vi "Convert Binary to TSV.vi"(8 "This VI":refnum<vi>, 11 "TDMS DataFile Name":path) -> ()   [LabVIEW 2023]
uses:
  User_Vi/Settings.vi
panel:
  out "error out 2":errorcluster
  out "error out":errorcluster
  out "Save a copy of the Binary Data File":bool
  out "PointsPerRow":u64
  out "NumberOfRowstoSave":i16
  out "ApproxBytes":dbl
  out "Save File Path":path
  out "Save Channels Separatly":bool
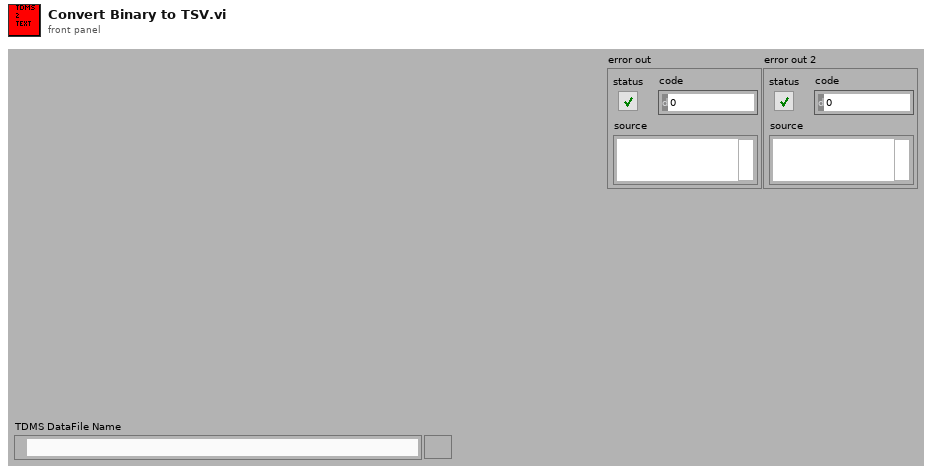
[diagram p1: front panel]
types:
  T1 = enum16{"open", "open or create", "create or replace", "create", "open (read-only)"}
  T2 = enum16{"open", "replace", "create", "open or create", "replace or create", "replace or create with confirmation"}
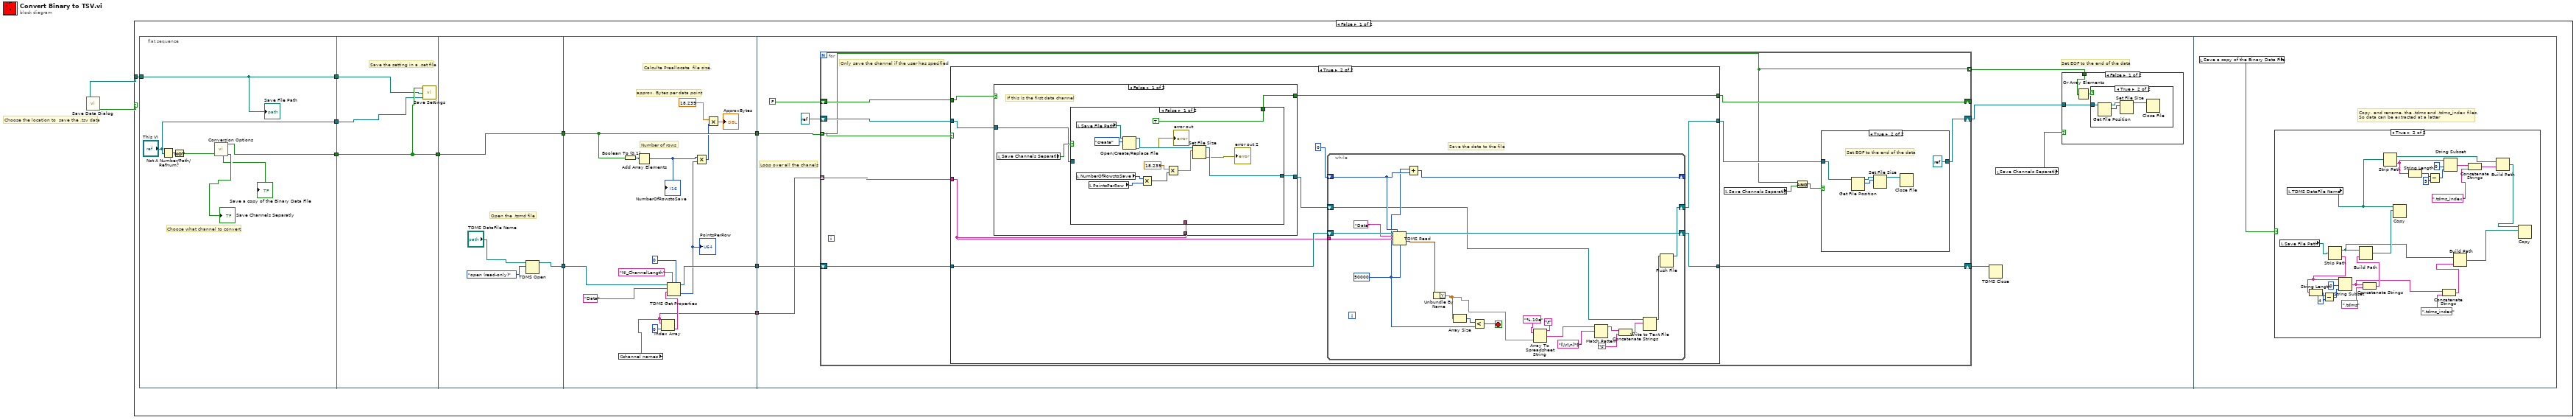
[diagram p0: block diagram]
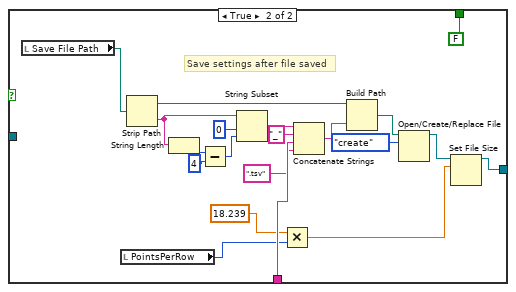
[diagram p6: hidden frame]
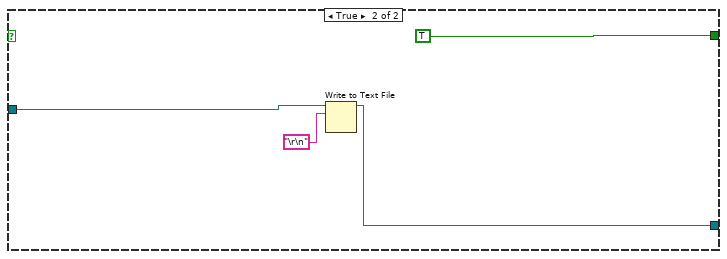
[diagram p7: hidden frame]
diagram:
  # "Choose the location to  save the .tsv data"
  n1 = call "Save Data Dialog.vi"() -> ("cancelled"=w1:bool, "selected path"=w2:path)  [unwired: 1 in]
  n2 = case shown="False" w1 {
    tunnel: w2 -> [w12 _]
    frame False {
      n3 = flat-sequence {
        tunnel: w12 -> [w17]
        tunnel: [w17] -> w7
        tunnel: [w19] -> w5
        tunnel: ["This VI"] -> w4
        tunnel: w7 -> [w21]
        tunnel: [w22] -> w6
        tunnel: w5 -> [w22]
        tunnel: w4 -> [w20]
        tunnel: [w24] -> w11
        tunnel: [w25] -> w8
        tunnel: w6 -> [w24]
        tunnel: w11 -> [w41]
        tunnel: [w41] -> w10
        tunnel: [w36] -> w9
        tunnel: w8 -> [w39]
        tunnel: [w27] -> w3
        tunnel: w10 -> [w50]
        tunnel: w9 -> [w48]
        tunnel: w3 -> [w43]
        frame #0 {
          # "Choose what channel to convert"
          n4 = Not A Number/Path/Refnum?(number/path/refnum="This VI") -> (NaN/Path/Refnum?=w15:bool)
          n5 = Not(x=w15) -> (.not. x?=w13:bool)
          n6 = call "Conversion Options.vi"("Save a copy of the Binary Data File"=w13) -> ("Save Each Channel as a Separate File indicator"=→"Save Channels Separatly":bool, "Array"=w19:bool[], "Save a copy of the Binary Data File"=→"Save a copy of the Binary Data File":bool)  [unwired: 8 in]
          "Save File Path" <- w17
        }
        frame #1 {
          # "Save the setting in a .set file"
          n7 = call "Save Settings.vi"("This VI"=w20, "Path"=w21, "Array"=w22) -> ()  [unwired: 1 in]
        }
        frame #2 {
          # "Open the .tsmd file"
          n8 = TDMS Open(10:T1."open (read-only)" ("operation (0:open)"), 11:"TDMS DataFile Name") -> (3:w25:refnum<k34>)  [unwired: 5 in, 1 out]
        }
        frame #3 {
          # "approx. Bytes per data point"
          # "Number of rows"
          # "Calculte Preallocate  file size."
          n9 = global read "Settings.vi" "channel names"() -> (w27:string[])
          n10 = Boolean To (0,1)(Boolean=w41) -> (0, 1=w40:i16[])
          n11 = Add Array Elements(numeric array=w40) -> (sum=w33:i16)
          "NumberOfRowstoSave" <- w33
          n12 = Index Array(array=w27, index=0) -> (element=w28:string)
          n13 = TDMS Get Properties(5:u64 0, 7:"NI_ChannelLength" ("property name"), 9:w28, 10:"Data" ("group name in"), 11:w39) -> (3:w36:refnum<k34>, 4:w34:u64)  [unwired: 1 in, 4 out]
          "PointsPerRow" <- w34
          n14 = Multiply(x=w33, y=w34) -> (x*y=w32:u64)
          n15 = Multiply(x=18.239, y=w32) -> (x*y=→"ApproxBytes":dbl)
        }
        frame #4 {
          # "Loop over all the chanels"
          # "Set EOF to the end of the data"
          n16 = for {
            tunnel: w50 -> [w58] mode=indexing
            shift-right: [w67] -> _
            shift-left: FALSE -> [w68]
            tunnel: w43 -> [w66] mode=indexing
            shift-right: [w61] -> w46
            shift-left: refnum<file> refnum ("refnum out") -> [w65]
            shift-right: [w63] -> w47
            shift-left: w48 -> [w64]
            tunnel: [w58] -> w42 mode=indexing
            # "Only save the channel if the user has specified"
            n17 = case shown="True" w58 {
              tunnel: w66 -> [_ w78]
              tunnel: w68 -> [w77 w86]
              tunnel: [w77 w79] -> w67
              tunnel: [w76 w82] -> w62
              tunnel: w65 -> [w76 w85]
              tunnel: w64 -> [w75 w81]
              tunnel: [w75 w80] -> w63
              frame False {
              }
              frame True {
                # "Save the data to the file"
                n18 = case shown="False" w86 {
                  tunnel: w85 -> [w111 w148]
                  tunnel: [w110 w147] -> w83
                  tunnel: [w109 TRUE] -> w79
                  tunnel: w78 -> [w108 _]
                  frame False {
                    # "If this is the first data channel"
                    n19 = local read "Save Channels Separatly"() -> (w112:bool)
                    n20 = case shown="False" w112 {
                      tunnel: w111 -> [_ _]
                      tunnel: [w121 w125] -> w110
                      tunnel: [TRUE FALSE] -> w109
                      tunnel: w108 -> [_ w133]
                      frame False {
                        n21 = local read "NumberOfRowstoSave"() -> (w119:i16)
                        n22 = local read "Save File Path"() -> (w123:path)
                        n23 = local read "PointsPerRow"() -> (w118:u64)
                        n24 = Open/Create/Replace File(file path (use dialog)=w123, operation (0:open)=T2."create") -> (refnum out=w122:refnum<file>, error out=→"error out":errorcluster)  [unwired: 4 in, 1 out]
                        n25 = Multiply(x=w119, y=w118) -> (x*y=w117:u64)
                        n26 = Multiply(x=18.239, y=w117) -> (x*y=w115:dbl)
                        n27 = Set File Size(6:w115, 7:w122) -> (0:→"error out 2":errorcluster, 3:w121:refnum<file>)  [unwired: 1 in]
                      }
                      frame True {
                        # "Save settings after file saved"
                        n28 = local read "Save File Path"() -> (w135:path)
                        n29 = local read "PointsPerRow"() -> (w128:u64)
                        n30 = Strip Path(path=w135) -> (stripped path=w136:path, name=w140:string)
                        n31 = String Length(string=w140) -> (length=w141:i32)
                        n32 = Subtract(x=w141, y=4) -> (x-y=w142:i32)
                        n33 = String Subset(string=w140, offset (0)=0, length (rest)=w142) -> (substring=w138:string)
                        n34 = Multiply(x=18.239, y=w128) -> (x*y=w126:dbl)
                        n35 = Concatenate Strings(w138, "_" ("string"), w133, ".tsv") -> (w137:string)
                        n36 = Build Path(base path=w136, name or relative path=w137) -> (appended path=w129:path)
                        n37 = Open/Create/Replace File(file path (use dialog)=w129, operation (0:open)=T2."create") -> (refnum out=w130:refnum<file>)  [unwired: 4 in, 2 out]
                        n38 = Set File Size(6:w126, 7:w130) -> (3:w125:refnum<file>)  [unwired: 1 in, 1 out]
                      }
                    }
                  }
                  frame True {
                    n39 = Write to Text File(file (use dialog)=w148, text="\r\n") -> (refnum out=w147:refnum<file>)  [unwired: 2 in, 2 out]
                  }
                }
                n40 = while {
                  tunnel: w78 -> [w107]
                  shift-right: [w105] -> w80
                  shift-left: w81 -> [w106]
                  shift-right: [w102] -> w82
                  shift-left: w83 -> [w89]
                  shift-right: [w104] -> _
                  shift-left: i64 0 ("offset (0)") -> [w103]
                  stop <- w99 stop-if-true
                  w97 = i64 50000 ("count (-1: all)")
                  n41 = TDMS Read(0:w106, 1:w103, 2:w97, 5:"Data" ("group name in"), 7:w107) -> (4:w105:refnum<k34>, 10:w100:waveform(dbl))  [unwired: 3 in, 4 out]
                  n42 = Add(x=w97, y=w103) -> (x+y=w104:i64)
                  n43 = Unbundle By Name(w100) -> ("Y"=w94:dbl[])
                  n44 = Array Size(array=w94) -> (size(s)=w98:i32)
                  n45 = Less?(x=w98, y=w97) -> (x < y?=w99:bool)
                  n46 = Array To Spreadsheet String(delimiter (Tab)="\t", array=w94, 3:"%.10e") -> (spreadsheet string=w91:string)
                  n47 = Match Pattern(string=w91, regular expression="[\\r\\n]*$") -> (before substring=w92:string)  [unwired: 1 in, 3 out]
                  n48 = Concatenate Strings(w92, "\t") -> (w88:string)
                  n49 = Write to Text File(file (use dialog)=w89, text=w88) -> (refnum out=w87:refnum<file>)  [unwired: 2 in, 2 out]
                  n50 = Flush File(refnum=w87) -> (refnum out=w102:refnum<file>)  [unwired: 1 in, 1 out]
                }
              }
            }
            n51 = local read "Save Channels Separatly"() -> (w60:bool)
            n52 = And(x=w58, y=w60) -> (x .and. y?=w59:bool)
            n53 = case shown="True" w59 {
              tunnel: w62 -> [w69 w71]
              tunnel: [w69 refnum<file> refnum ("refnum out")] -> w61
              frame False {
              }
              frame True {
                # "Set EOF to the end of the data"
                n54 = Get File Position(7:w71) -> (2:w73:i64, 3:w72:refnum<file>)  [unwired: 1 in, 1 out]
                n55 = Set File Size(6:w73, 7:w72) -> (3:w74:refnum<file>)  [unwired: 1 in, 1 out]
                n56 = Close File(refnum=w74) -> ()  [unwired: 1 in, 2 out]
              }
            }
          }
          n57 = TDMS Close(11:w47) -> ()  [unwired: 1 in, 2 out]
          n58 = local read "Save Channels Separatly"() -> (w44:bool)
          n59 = case shown="False" w44 {
            tunnel: w46 -> [w53 _]
            tunnel: w42 -> [w52 _]
            frame False {
              n60 = Or Array Elements(Boolean array=w52) -> (logical OR=w51:bool)
              n61 = case shown="True" w51 {
                tunnel: w53 -> [_ w57]
                frame False {
                }
                frame True {
                  n62 = Get File Position(7:w57) -> (2:w55:i64, 3:w56:refnum<file>)  [unwired: 1 in, 1 out]
                  n63 = Set File Size(6:w55, 7:w56) -> (3:w54:refnum<file>)  [unwired: 1 in, 1 out]
                  n64 = Close File(refnum=w54) -> ()  [unwired: 1 in, 2 out]
                }
              }
            }
            frame True {
            }
          }
        }
        frame #5 {
          # "Copy, and rename, the .tdms and .tdms_index files.\nSo data can be extracted at a latter"
          n65 = local read "Save a copy of the Binary Data File"() -> (w149:bool)
          n66 = case shown="True" w149 {
            frame False {
            }
            frame True {
              n67 = local read "Save File Path"() -> (w174:path)
              n68 = local read "TDMS DataFile Name"() -> (w160:path)
              n69 = Strip Path(path=w174) -> (stripped path=w163:path, name=w168:string)
              n70 = String Length(string=w168) -> (length=w171:i32)
              n71 = Subtract(x=w171, y=4) -> (x-y=w170:i32)
              n72 = String Subset(string=w168, offset (0)=0, length (rest)=w170) -> (substring=w162:string)
              n73 = Concatenate Strings(w162, ".tdms") -> (w166:string)
              n74 = Build Path(base path=w163, name or relative path=w166) -> (appended path=w173:path)
              n75 = Strip Path(path=w160) -> (stripped path=w151:path, name=w154:string)
              n76 = Copy(10:w173, 11:w160) -> ()  [unwired: 3 in, 3 out]
              n77 = String Length(string=w154) -> (length=w156:i32)
              n78 = Subtract(x=w156, y=5) -> (x-y=w157:i32)
              n79 = Concatenate Strings(w162, ".tdms_index") -> (w165:string)
              n80 = String Subset(string=w154, offset (0)=0, length (rest)=w157) -> (substring=w159:string)
              n81 = Build Path(base path=w163, name or relative path=w165) -> (appended path=w161:path)
              n82 = Concatenate Strings(w159, ".tdms_index") -> (w152:string)
              n83 = Build Path(base path=w151, name or relative path=w152) -> (appended path=w150:path)
              n84 = Copy(10:w161, 11:w150) -> ()  [unwired: 3 in, 3 out]
            }
          }
        }
      }
    }
    frame True {
    }
  }
